vi "PID-Ctrl.vi"() -> (3 ".not. x?":bool)   [LabVIEW 2011]
uses:
  <vilib>/Analysis/2dsp.llb/Integral Method.ctl
  <vilib>/Analysis/NI_AALPro.lvlib
  <vilib>/Analysis/NI_AALBase.lvlib
panel:
  in  "stop":bool
  out "pause":bool
  in  "X time Off":dbl
  out "tempo":dbl[](array[numeric])
  out "milisec 2":dbl
  in  "fator Ganho":dbl=1.0
  out "milisec":dbl
  out "tempo 2":dbl[](array[numeric])
  out "ON/OFF":bool
  out "t-on":dbl
  out "t-PID":bool
  in  "time (s) Loop":dbl
  out "PID limit":bool
  in  "PID limit":dbl
  in  "PID-ON/OFF":bool
  out "D-mean":dbl format="%0.2f"
  out "I-mean":dbl format="%0.2f"
  out "Ganho":dbl
  in  "Kd(s)":dbl(slide) scale=0.0..10.0
  in  "Ki(s)":dbl(slide) scale=0.0..10.0
  in  "Kp":dbl(slide) scale=0.0..10.0
  in  "D (Td)":bool
  in  "I (Ti)":bool
  in  "PID":bool
  in  "T - ON/OFF":bool
  out "intrp- T":dbl format="%0.2f"
  out "output array":dbl[][](array[numeric])
  in  "Ndata":i32
  in  "New Button":bool
  in  "SP":dbl(slide) scale=0.0..150.0
  out "Waveform T":dynamicdata(graph)
  out "ThermC":dbl(slide) scale=0.0..150.0
  out "min":dbl
  out "Max":dbl
  in  "PIDmin":dbl
  in  "PIDMax":dbl
  # "PID controller"
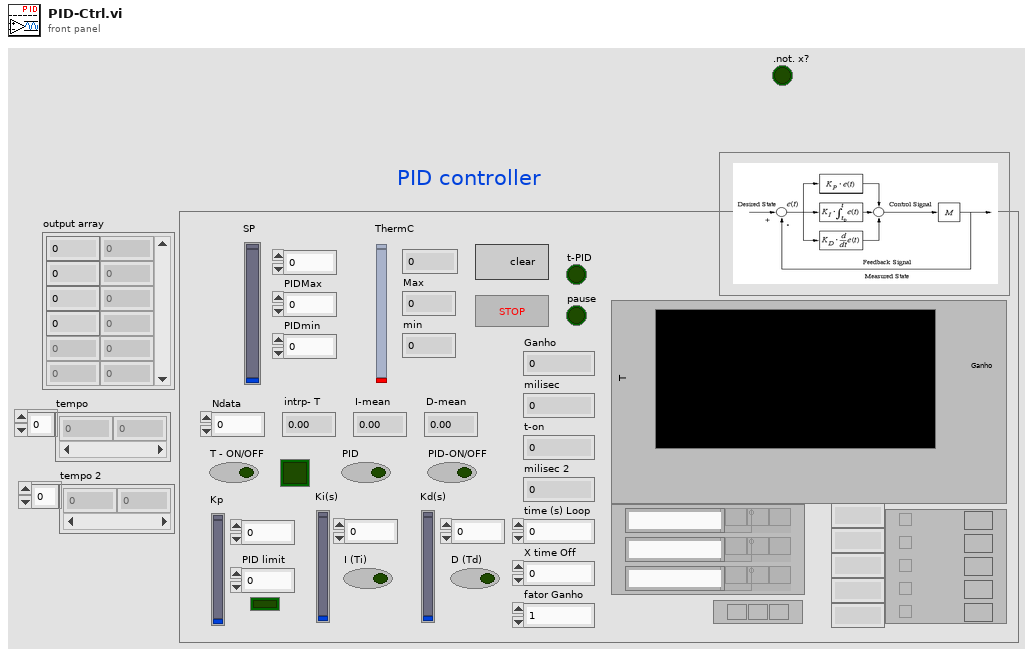
[diagram p1: front panel]
types:
  T1 = enum16{"Linear", "Polynomial", "Spline", "Rational"}
  T2 = cluster{"Type of Interpolation":enum16{"Linear", "Polynomial", "Spline", "Rational"}, "Points Between":i32}
  T3 = typedef "NI_AALPro.lvlib/Integral Method.ctl" = i32
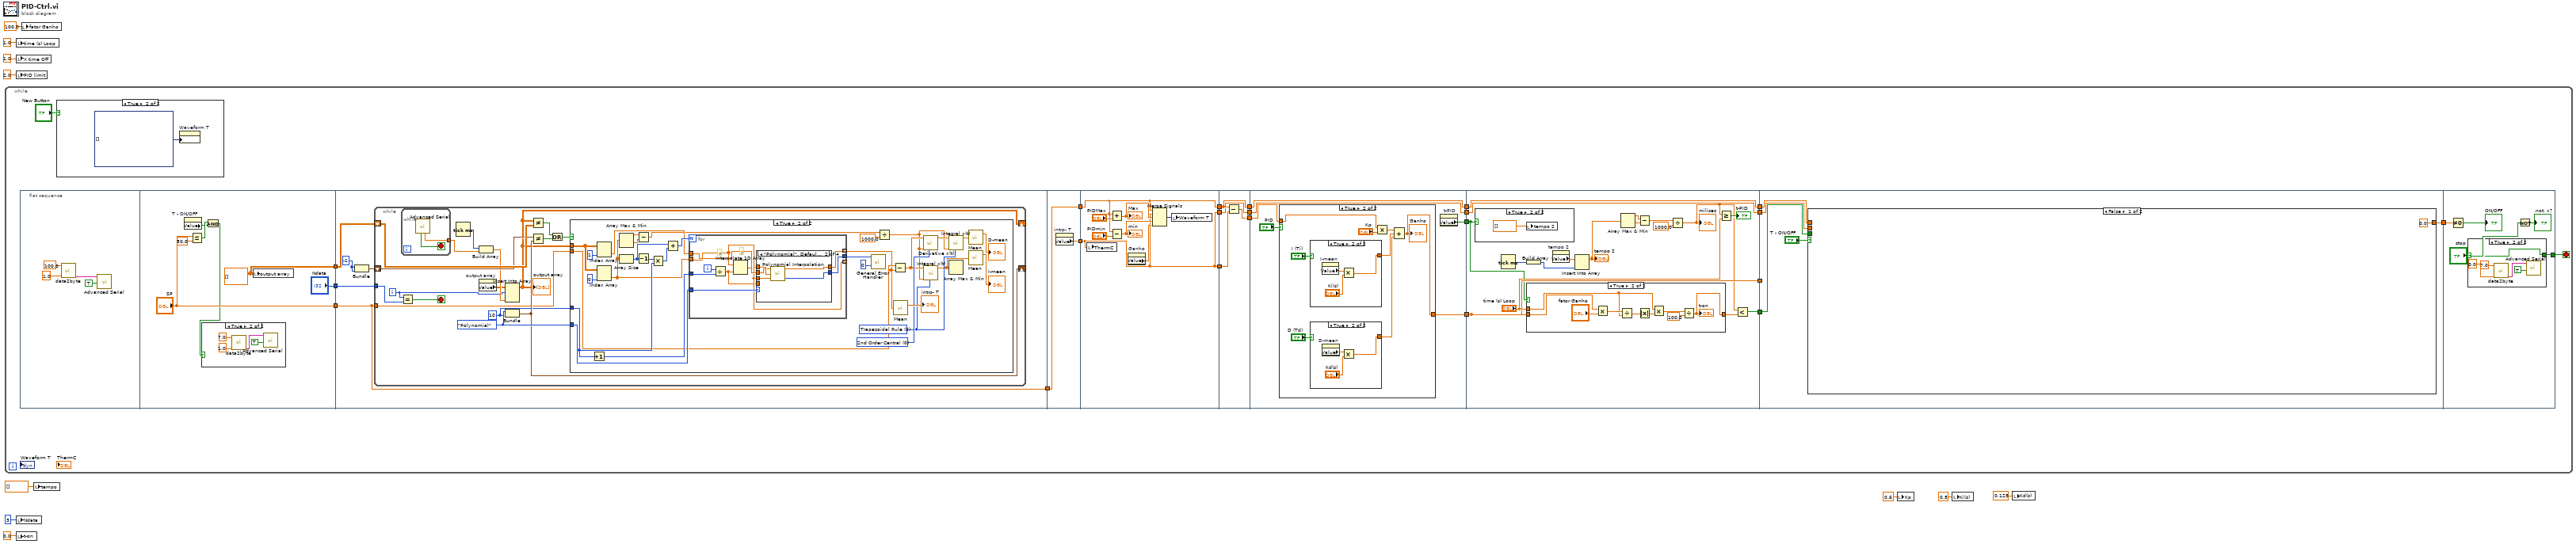
[diagram p0: block diagram]
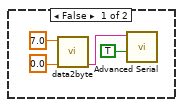
[diagram p3: hidden frame]
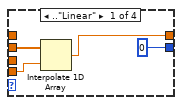
[diagram p5: hidden frame]
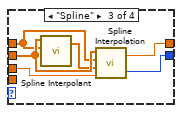
[diagram p6: hidden frame]
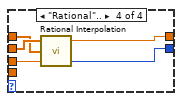
[diagram p7: hidden frame]
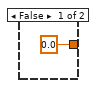
[diagram p8: hidden frame]
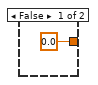
[diagram p9: hidden frame]
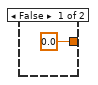
[diagram p10: hidden frame]
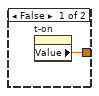
[diagram p12: hidden frame]
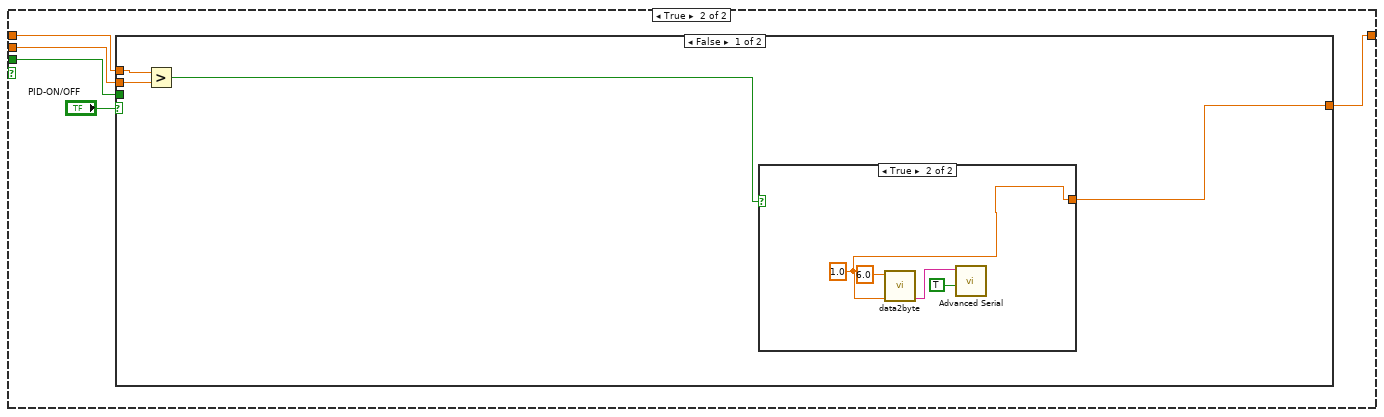
[diagram p13: hidden frame]
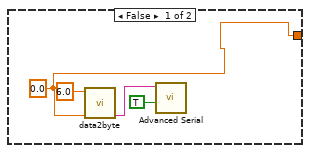
[diagram p14: hidden frame]
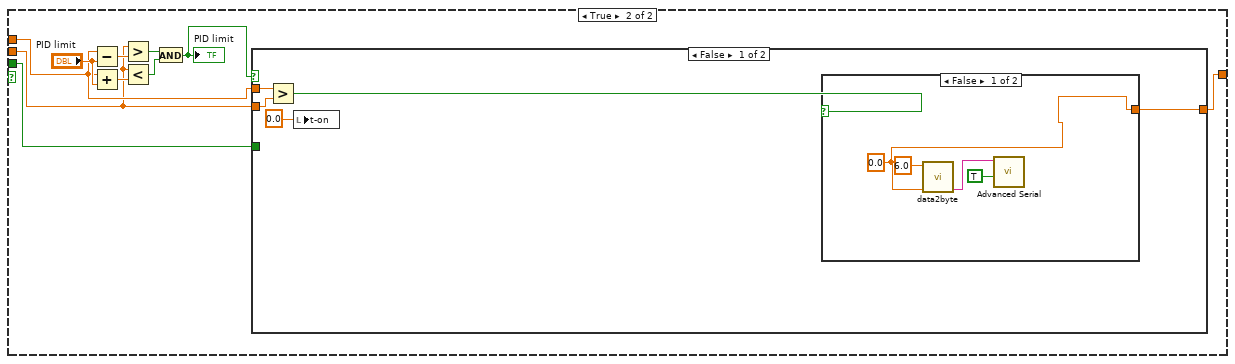
[diagram p15: hidden frame]
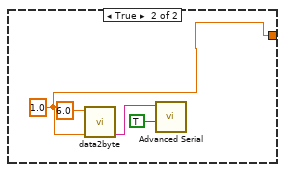
[diagram p16: hidden frame]
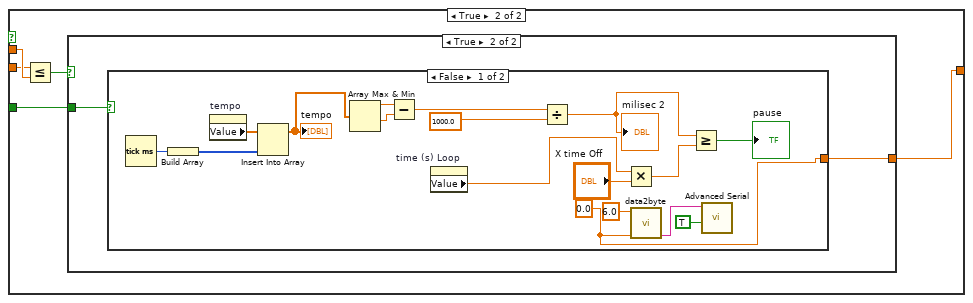
[diagram p17: hidden frame]
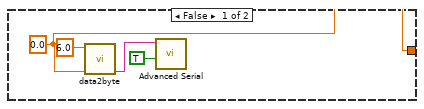
[diagram p18: hidden frame]
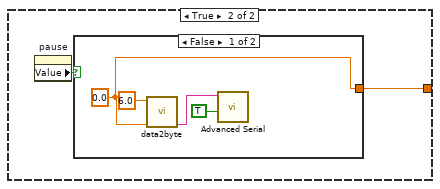
[diagram p19: hidden frame]
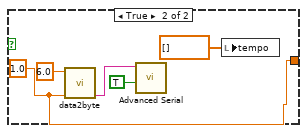
[diagram p20: hidden frame]
diagram:
  n1 = while {
    stop <- w11 stop-if-true
    n2 = flat-sequence {
      tunnel: ["SP"] -> w33
      tunnel: ["Ndata"] -> w32
      tunnel: [w44] -> w31
      tunnel: w33 -> [w54]
      tunnel: [w54] -> w30
      tunnel: w32 -> [w56]
      tunnel: w31 -> [w55]
      tunnel: w30 -> [w138]
      tunnel: [w138] -> w29
      tunnel: [w137] -> w28
      tunnel: w29 -> [w141]
      tunnel: w28 -> [w140]
      tunnel: [w140] -> w26
      tunnel: [w141] -> w25
      tunnel: [w140] -> w13
      tunnel: w26 -> [w149]
      tunnel: w25 -> [w148]
      tunnel: [w148] -> w18
      tunnel: [w150] -> w17
      tunnel: [w147] -> w14
      tunnel: w13 -> [w147]
      tunnel: w18 -> [w156]
      tunnel: [w156] -> w24
      tunnel: w17 -> [w154]
      tunnel: [w153] -> w22
      tunnel: [w152] -> w19
      tunnel: [w151] -> w15
      tunnel: w14 -> [w151]
      tunnel: w24 -> [w190]
      tunnel: [w190] -> w23
      tunnel: w22 -> [w186]
      tunnel: [w186] -> w21
      tunnel: [w185] -> w20
      tunnel: w19 -> [w175]
      tunnel: [w174] -> w16
      tunnel: w15 -> [w174]
      tunnel: w23 -> [w205]
      tunnel: w21 -> [_]
      tunnel: w20 -> [w204]
      tunnel: w16 -> [w203]
      tunnel: [w202] -> w12
      tunnel: w12 -> [w290]
      tunnel: [w289] -> w11
      frame #0 {
        n3 = call "data2byte.vi"("argument"=1.0 ("number"), "new function"=100.0) -> ("protocol"=w35:string)  [unwired: 8 in, 1 out]
        n4 = call "Advanced Serial.vi"("Write"=TRUE ("write"), "string to write"=w35) -> ()  [unwired: 3 in, 7 out]
      }
      frame #1 {
        w44 = dbl[][] [] ("Array 2")
        n5 = property on="T - ON/OFF" class="Bool (strict)"() -> ("Value"=w40:bool)  [unwired: 2 in, 2 out]
        n6 = Less Or Equal?(x="SP", y=50.0) -> (x <= y?=w41:bool)
        n7 = And(x=w41, y=w40) -> (x .and. y?=w39:bool)
        n8 = case shown="True" w39 {
          frame False {
            n9 = call "data2byte.vi"("argument"=0.0 ("number"), "new function"=7.0) -> ("protocol"=w46:string)  [unwired: 8 in, 1 out]
            n10 = call "Advanced Serial.vi"("Write"=TRUE ("write"), "string to write"=w46) -> ()  [unwired: 3 in, 7 out]
          }
          frame True {
            n11 = call "data2byte.vi"("argument"=1.0 ("number"), "new function"=7.0) -> ("protocol"=w50:string)  [unwired: 8 in, 1 out]
            n12 = call "Advanced Serial.vi"("Write"=TRUE ("write"), "string to write"=w50) -> ()  [unwired: 3 in, 7 out]
          }
        }
        n13 = local write "output array"(w44) -> ()
      }
      frame #2 {
        w57 = -1
        n14 = Bundle(w57, w57) -> (w58:cluster{i32, i32})  [unwired: 1 in]
        n15 = while {
          shift-left: w58 -> [w70]
          shift-right: [w69] -> _
          shift-left: w55 -> [w75]
          shift-right: [w66] -> _
          tunnel: w56 -> [w63]
          tunnel: w54 -> [w61]
          i -> [w62]
          stop <- w64 stop-if-true
          w68 = 10 ("Points Between")
          w71 = T1."Polynomial" ("Type of Interpolation")
          n16 = Equal?(x=w62, y=w63) -> (x = y?=w64:bool)
          n17 = while {
            tunnel: [w76] -> w59
            stop <- w77 stop-if-true
            n18 = call "Advanced Serial.vi"() -> ("RTD-chamber (ºC)"=w76:sgl, "32bytes"=w77:bool)  [unwired: 5 in, 5 out]
          }
          n19 = Tick Count (ms)() -> (millisecond timer value=w60:u32)
          n20 = Build Array(w60, w59) -> (w67:sgl[])
          n21 = property on="output array" class="Arr (strict)"() -> ("Value"=w65:dbl[][])  [unwired: 2 in, 2 out]
          n22 = Insert Into Array(array=w65, index (row)=w62, new element=w67) -> (w66:dbl[][])  [unwired: 1 in]
          "output array" <- w66
          n23 = Bundle("Type of Interpolation"=w71, "Points Between"=w68) -> (w69:T2)  [unwired: 1 in]
          n24 = Not Equal?(x=w66, y=w75) -> (x != y?=w74:bool)
          n25 = Not Equal?(x=w70, y=w69) -> (x != y?=w73:bool)
          n26 = Or(x=w74, y=w73) -> (x .or. y?=w72:bool)
          n27 = case shown="True" w72 {
            tunnel: w66 -> [_ w103]
            tunnel: w71 -> [_ w97]
            tunnel: w68 -> [_ w96]
            tunnel: w61 -> [_ w93]
            frame False {
            }
            frame True {
              w88 = T3 0 items=["Trapezoidal Rule", "Simpson's Rule", "Simpson's 3/8 Rule", "Bode Rule"] ("integration method")
              w94 = u16 0 items=["2nd Order Central", "4th Order Central", "Forward", "Backward"] ("method")
              n28 = Increment(x=w96) -> (x+1=w101:i32)
              n29 = Index Array(array=w103, index (col)=1) -> (element=w82:dbl[])  [unwired: 1 in]
              n30 = Index Array(array=w103, index (col)=0) -> (element=w87:dbl[])  [unwired: 1 in]
              n31 = Array Max & Min(array=w87) -> (max value=w91:dbl, min value=w90:dbl)  [unwired: 2 out]
              n32 = Array Size(array=w87) -> (size(s)=w99:i32)
              n33 = Subtract(x=w91, y=w90) -> (x-y=w80:dbl)
              n34 = Decrement(x=w99) -> (x-1=w102:i32)
              n35 = Multiply(x=w102, y=w96) -> (x*y=w100:i32)
              n36 = Add(x=w99, y=w100) -> (x+y=w98:i32)
              n37 = for {
                N: w98 -> [_]
                tunnel: w82 -> [w116]
                tunnel: w87 -> [w110]
                tunnel: [w115] -> w107
                tunnel: w97 -> [w111]
                tunnel: w101 -> [w113]
                tunnel: [w112] -> w78 mode=indexing
                tunnel: [w109] -> _ mode=indexing
                i -> [w114]
                # "x"
                # "y"
                n38 = Divide(x=w114, y=w113) -> (x/y=w108:dbl)
                n39 = Interpolate 1D Array(1:w108, 2:w110) -> (0:w109:dbl)
                n40 = case shown="\"Polynomial\", Default" w111 {
                  tunnel: w109 -> [_ w125 w128 w132]
                  tunnel: [w119 w124 w126 w134] -> w112
                  tunnel: [0 w123 w127 w133] -> w115
                  tunnel: w110 -> [_ w122 w129 w135]
                  tunnel: w116 -> [w120 w121 w131 w136]
                  tunnel: w108 -> [w117 _ _ _]
                  frame .."Linear" {
                    n41 = Interpolate 1D Array(1:w117, 2:w120) -> (0:w119:dbl)
                  }
                  frame "Polynomial", Default {
                    n42 = call <vilib>:"Polynomial Interpolation.vi"("x value"=w125, "X"=w122, "Y"=w121) -> ("error"=w123:i32, "interpolation value"=w124:dbl)  [unwired: 1 out]
                  }
                  frame "Spline" {
                    n43 = call <vilib>:"Spline Interpolant.vi"("X"=w129, "Y"=w131) -> ("Interpolant"=w130:dbl[])  [unwired: 2 in, 1 out]
                    n44 = call <vilib>:"Spline Interpolation.vi"("x value"=w128, "Interpolant"=w130, "X"=w129, "Y"=w131) -> ("error"=w127:i32, "interpolation value"=w126:dbl)
                  }
                  frame "Rational".. {
                    n45 = call <vilib>:"Rational Interpolation.vi"("x value"=w132, "X"=w135, "Y"=w136) -> ("error"=w133:i32, "interpolation value"=w134:dbl)  [unwired: 1 out]
                  }
                }
              }
              n46 = call <vilib>:"General Error Handler.vi"("[error code] (0)"=w107, "type of dialog (OK msg:1)"=0) -> ()  [unwired: 9 in, 5 out]
              n47 = Divide(x=w80, y=1000.0) -> (x/y=w79:dbl)
              n48 = Subtract(x=w93, y=w78) -> (x-y=w92:dbl[])
              n49 = call <vilib>:"Mean.vi"("X"=w78) -> ("mean"=→"intrp- T":dbl)  [unwired: 1 out]
              n50 = call <vilib>:"Derivative x(t).vi"("method"=w94, "dt"=w79, "X"=w92) -> ("dX/dt"=w89:dbl[])  [unwired: 7 in, 1 out]
              n51 = call <vilib>:"Integral x(t).vi"("integration method"=w88, "dt"=w79, "X"=w92) -> ("Integral X"=w83:dbl[])  [unwired: 7 in, 1 out]
              n52 = call <vilib>:"Integral x(t).vi"("integration method"=w88, "dt"=w79, "X"=w89) -> ("Integral X"=w86:dbl[])  [unwired: 7 in, 1 out]
              n53 = Array Max & Min(array=w83) -> ()  [unwired: 4 out]
              n54 = call <vilib>:"Mean.vi"("X"=w86) -> ("mean"=→"D-mean":dbl)  [unwired: 1 out]
              n55 = call <vilib>:"Mean.vi"("X"=w83) -> ("mean"=→"I-mean":dbl)  [unwired: 1 out]
            }
          }
        }
      }
      frame #3 {
        n56 = property on="intrp- T" class="DigNum (strict)"() -> ("Value"=w137:dbl)  [unwired: 2 in, 2 out]
      }
      frame #4 {
        n57 = local write "ThermC"(w140) -> ()
        n58 = Add(x=w141, y="PIDMax") -> (x+y=w142:dbl)
        "Max" <- w142
        n59 = Subtract(x=w141, y="PIDmin") -> (x-y=w143:dbl)
        "min" <- w143
        n60 = property on="Ganho" class="DigNum (strict)"() -> ("Value"=w139:dbl)  [unwired: 2 in, 2 out]
        n61 = Merge Signals(w141, w140, w142, w143, w139) -> (w144:dynamicdata)
        n62 = local write "Waveform T"(w144) -> ()
      }
      frame #5 {
        n63 = Subtract(x=w148, y=w149) -> (x-y=w150:dbl)
      }
      frame #6 {
        n64 = case shown="True" "PID" {
          tunnel: w154 -> [_ w159]
          tunnel: [0.0 w158] -> w153
          frame False {
          }
          frame True {
            n65 = case shown="True" "I (Ti)" {
              tunnel: [0.0 w173] -> w161
              frame False {
              }
              frame True {
                n66 = property on="I-mean" class="DigNum (strict)"() -> ("Value"=w171:dbl)  [unwired: 2 in, 2 out]
                n67 = Multiply(x=w171, y="Ki(s)") -> (x*y=w173:dbl)
              }
            }
            n68 = case shown="True" "D (Td)" {
              tunnel: [0.0 w169] -> w160
              frame False {
              }
              frame True {
                n69 = property on="D-mean" class="DigNum (strict)"() -> ("Value"=w167:dbl)  [unwired: 2 in, 2 out]
                n70 = Multiply(x=w167, y="Kd(s)") -> (x*y=w169:dbl)
              }
            }
            n71 = Multiply(x=w159, y="Kp") -> (x*y=w162:dbl)
            n72 = Compound Arithmetic op=ADD(w162, w161, w160) -> (w158:dbl)
            "Ganho" <- w158
          }
        }
        n73 = property on="t-PID" class="Bool (strict)"() -> ("Value"=w152:bool)  [unwired: 2 in, 2 out]
      }
      frame #7 {
        n74 = case shown="True" w175 {
          frame False {
          }
          frame True {
            n75 = local write "tempo 2"(dbl[] [] ("Time")) -> ()
          }
        }
        n76 = Tick Count (ms)() -> (millisecond timer value=w182:u32)
        n77 = Build Array(w182) -> (w183:u32[])
        n78 = case shown="True" w175 {
          tunnel: w186 -> [_ w201]
          tunnel: "time (s) Loop" -> [_ w198]
          tunnel: [w192 w195] -> w187
          frame False {
            n79 = property on="t-on" class="DigNum (strict)"() -> ("Value"=w192:dbl)  [unwired: 2 in, 2 out]
          }
          frame True {
            n80 = Multiply(x=w201, y="fator Ganho") -> (x*y=w200:dbl)
            n81 = Divide(x=w200, y=w198) -> (x/y=w199:dbl)
            n82 = Absolute Value(x=w199) -> (abs(x)=w197:dbl)
            n83 = Multiply(x=w198, y=w197) -> (x*y=w196:dbl)
            n84 = Divide(x=w196, y=100.0) -> (x/y=w195:dbl)
            "t-on" <- w195
          }
        }
        n85 = property on="tempo 2" class="Arr (strict)"() -> ("Value"=w184:dbl[])  [unwired: 2 in, 2 out]
        n86 = Insert Into Array(array=w184, new element=w183) -> (w181:dbl[])  [unwired: 1 in]
        "tempo 2" <- w181
        n87 = Array Max & Min(array=w181) -> (max value=w180:dbl, min value=w179:dbl)  [unwired: 2 out]
        n88 = Subtract(x=w180, y=w179) -> (x-y=w178:dbl)
        n89 = Divide(x=w178, y=1000.0) -> (x/y=w176:dbl)
        "milisec" <- w176
        n90 = Greater Or Equal?(x=w176, y="time (s) Loop") -> (x >= y?=→"t-PID":bool)
        n91 = Less?(x=w176, y=w187) -> (x < y?=w185:bool)
      }
      frame #8 {
        n92 = case shown="False" "T - ON/OFF" {
          tunnel: w205 -> [_ w211]
          tunnel: w204 -> [_ w210]
          tunnel: w203 -> [_ w209]
          tunnel: [0.0 ("number") w208] -> w202
          frame False {
          }
          frame True {
            n93 = case shown="False" "PID-ON/OFF" {
              tunnel: w211 -> [w216 w233]
              tunnel: w210 -> [_ w227]
              tunnel: w209 -> [w215 w226]
              tunnel: [w213 w225] -> w208
              frame False {
                n94 = Greater?(x=w216, y=w215) -> (0:w214:bool)
                n95 = case shown="True" w214 {
                  tunnel: [w217 w221] -> w213
                  frame False {
                    w217 = 0.0 ("number")
                    n96 = call "data2byte.vi"("argument"=w217, "new function"=6.0) -> ("protocol"=w218:string)  [unwired: 8 in, 1 out]
                    n97 = call "Advanced Serial.vi"("Write"=TRUE ("write"), "string to write"=w218) -> ()  [unwired: 3 in, 7 out]
                  }
                  frame True {
                    w221 = 1.0 ("number")
                    n98 = call "data2byte.vi"("argument"=w221, "new function"=6.0) -> ("protocol"=w222:string)  [unwired: 8 in, 1 out]
                    n99 = call "Advanced Serial.vi"("Write"=TRUE ("write"), "string to write"=w222) -> ()  [unwired: 3 in, 7 out]
                  }
                }
              }
              frame True {
                n100 = Subtract(x=w233, y="PID limit") -> (x-y=w229:dbl)
                n101 = Add(x=w233, y="PID limit") -> (x+y=w228:dbl)
                n102 = Greater?(x=w226, y=w229) -> (0:w231:bool)
                n103 = Less?(x=w226, y=w228) -> (x < y?=w230:bool)
                n104 = And(x=w231, y=w230) -> (x .and. y?=w232:bool)
                "PID limit" <- w232
                n105 = case shown="False" w232 {
                  tunnel: w233 -> [w238 w252]
                  tunnel: w227 -> [_ w251]
                  tunnel: w226 -> [w236 w249]
                  tunnel: [w235 w248] -> w225
                  frame False {
                    n106 = Greater?(x=w238, y=w236) -> (0:w239:bool)
                    n107 = local write "t-on"(0.0 ("%t-on")) -> ()
                    n108 = case shown="False" w239 {
                      tunnel: [w240 w244] -> w235
                      frame False {
                        w240 = 0.0 ("number")
                        n109 = call "data2byte.vi"("argument"=w240, "new function"=6.0) -> ("protocol"=w241:string)  [unwired: 8 in, 1 out]
                        n110 = call "Advanced Serial.vi"("Write"=TRUE ("write"), "string to write"=w241) -> ()  [unwired: 3 in, 7 out]
                      }
                      frame True {
                        w244 = 1.0 ("number")
                        n111 = call "data2byte.vi"("argument"=w244, "new function"=6.0) -> ("protocol"=w245:string)  [unwired: 8 in, 1 out]
                        n112 = call "Advanced Serial.vi"("Write"=TRUE ("write"), "string to write"=w245) -> ()  [unwired: 3 in, 7 out]
                      }
                    }
                  }
                  frame True {
                    n113 = Less Or Equal?(x=w249, y=w252) -> (x <= y?=w250:bool)
                    n114 = case shown="True" w250 {
                      tunnel: [w253 w257] -> w248
                      tunnel: w251 -> [_ w258]
                      frame False {
                        w253 = 0.0 ("number")
                        n115 = call "data2byte.vi"("argument"=w253, "new function"=6.0) -> ("protocol"=w254:string)  [unwired: 8 in, 1 out]
                        n116 = call "Advanced Serial.vi"("Write"=TRUE ("write"), "string to write"=w254) -> ()  [unwired: 3 in, 7 out]
                      }
                      frame True {
                        n117 = case shown="False" w258 {
                          tunnel: [w259 w277] -> w257
                          frame False {
                            w259 = 0.0 ("number")
                            n118 = Tick Count (ms)() -> (millisecond timer value=w266:u32)
                            n119 = Build Array(w266) -> (w265:u32[])
                            n120 = property on="tempo" class="Arr (strict)"() -> ("Value"=w264:dbl[])  [unwired: 2 in, 2 out]
                            n121 = Insert Into Array(array=w264, new element=w265) -> (w267:dbl[])  [unwired: 1 in]
                            "tempo" <- w267
                            n122 = Array Max & Min(array=w267) -> (max value=w268:dbl, min value=w269:dbl)  [unwired: 2 out]
                            n123 = Subtract(x=w268, y=w269) -> (x-y=w270:dbl)
                            n124 = property on="time (s) Loop" class="DigNum (strict)"() -> ("Value"=w274:dbl)  [unwired: 2 in, 2 out]
                            n125 = Divide(x=w270, y=1000.0) -> (x/y=w272:dbl)
                            "milisec 2" <- w272
                            n126 = Multiply(x=w274, y="X time Off") -> (x*y=w273:dbl)
                            n127 = call "data2byte.vi"("argument"=w259, "new function"=6.0) -> ("protocol"=w260:string)  [unwired: 8 in, 1 out]
                            n128 = Greater Or Equal?(x=w272, y=w273) -> (x >= y?=→"pause":bool)
                            n129 = call "Advanced Serial.vi"("Write"=TRUE ("write"), "string to write"=w260) -> ()  [unwired: 3 in, 7 out]
                          }
                          frame True {
                            n130 = property on="pause" class="Bool (strict)"() -> ("Value"=w276:bool)  [unwired: 2 in, 2 out]
                            n131 = case shown="False" w276 {
                              tunnel: [w278 w282] -> w277
                              frame False {
                                w278 = 0.0 ("number")
                                n132 = call "data2byte.vi"("argument"=w278, "new function"=6.0) -> ("protocol"=w279:string)  [unwired: 8 in, 1 out]
                                n133 = call "Advanced Serial.vi"("Write"=TRUE ("write"), "string to write"=w279) -> ()  [unwired: 3 in, 7 out]
                              }
                              frame True {
                                w282 = 1.0 ("number")
                                n134 = call "data2byte.vi"("argument"=w282, "new function"=6.0) -> ("protocol"=w283:string)  [unwired: 8 in, 1 out]
                                n135 = call "Advanced Serial.vi"("Write"=TRUE ("write"), "string to write"=w283) -> ()  [unwired: 3 in, 7 out]
                                n136 = local write "tempo"(dbl[] [] ("tempo")) -> ()
                              }
                            }
                          }
                        }
                      }
                    }
                  }
                }
              }
            }
          }
        }
      }
      frame #9 {
        n137 = Not Equal To 0?(x=w290) -> (x != 0?=→"ON/OFF":bool)
        n138 = case shown="True" "stop" {
          selector: "stop" -> [_ w297]
          tunnel: [FALSE w297] -> w289
          frame False {
          }
          frame True {
            n139 = call "data2byte.vi"("argument"=0.0 ("number"), "new function"=7.0) -> ("protocol"=w295:string)  [unwired: 8 in, 1 out]
            n140 = call "Advanced Serial.vi"("Write"=TRUE ("write"), "string to write"=w295) -> ()  [unwired: 3 in, 7 out]
          }
        }
        n141 = Not(x="stop") -> (.not. x?=→".not. x?":bool)
      }
    }
    n142 = case shown="True" "New Button" {
      frame False {
      }
      frame True {
        n143 = property on="Waveform T" class="WFChart (strict)"("History Data"=dynamicdata[] []) -> ()  [unwired: 2 in, 2 out]
      }
    }
  }
  n144 = local write "time (s) Loop"(1.0 ("time PID")) -> ()
  n145 = local write "X time Off"(1.0 ("X time Off")) -> ()
  n146 = local write "PID limit"(2.0 ("PID limit")) -> ()
  n147 = local write "Ndata"(3 ("Ndata")) -> ()
  n148 = local write "t-on"(0.0 ("%t-on")) -> ()
  n149 = local write "fator Ganho"(100.0 ("y")) -> ()
  n150 = local write "tempo"(dbl[] [] ("tempo")) -> ()
  n151 = local write "Kp"(0.6 ("Kp")) -> ()
  n152 = local write "Ki(s)"(0.5 ("Ki(s)")) -> ()
  n153 = local write "Kd(s)"(0.125 ("Kd(s)")) -> ()
